vi "Load Signal Bank 1.0.3 keh.vi"(7 "Transpose?":bool, 8 "error in (no error)":errorcluster, 9 "Input array":dbl[][](array[numeric]) format="%.2f", 10 "Active AO Array":u16[](array[numeric]), 11 "timeout (ms)":i32=5000) -> (0 "error out":errorcluster={"status"=FALSE, "code"=0, "source"="."}, 1 "Abort AO":bool, 3 "Time":i32)   [LabVIEW 2020]
uses:
  DAQ Engine VIs/PXI Globals.vi
panel:
  out "Waveform Graph":dbl[][](graph)
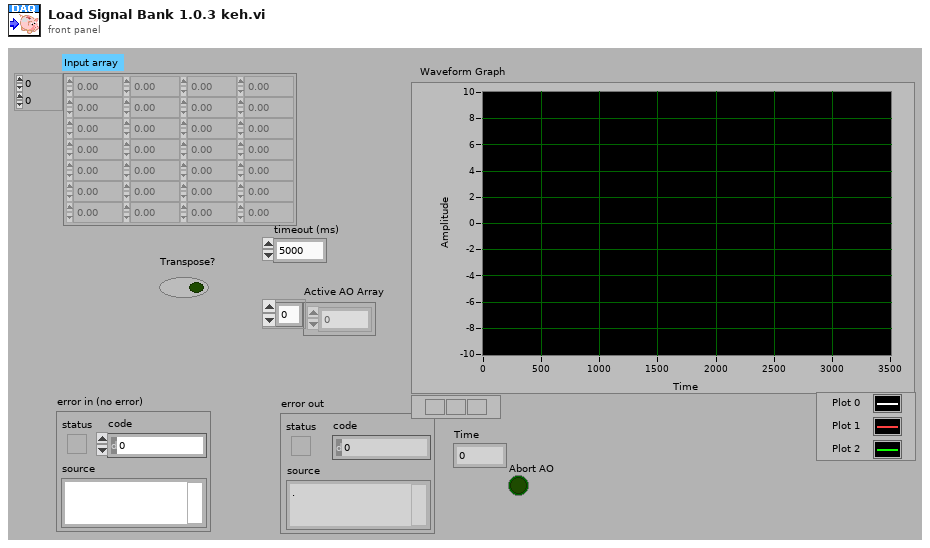
[diagram p1: front panel]
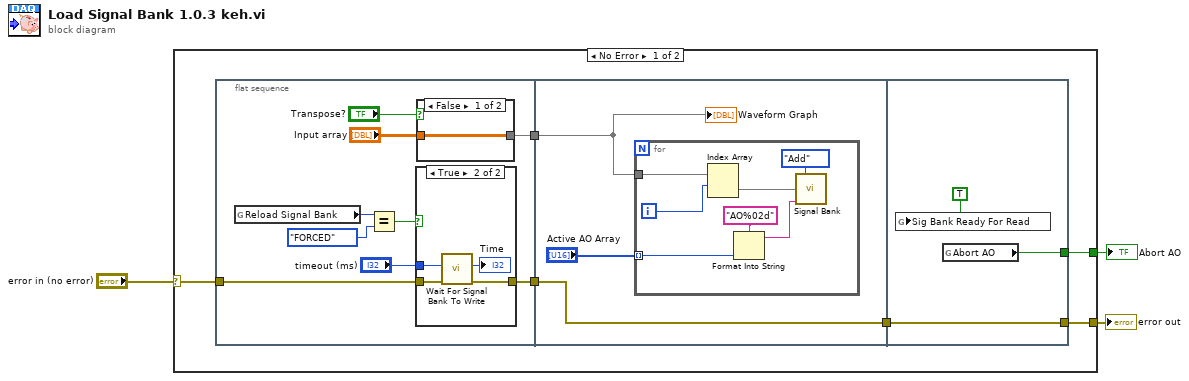
[diagram p0: block diagram]
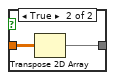
[diagram p2: hidden frame]
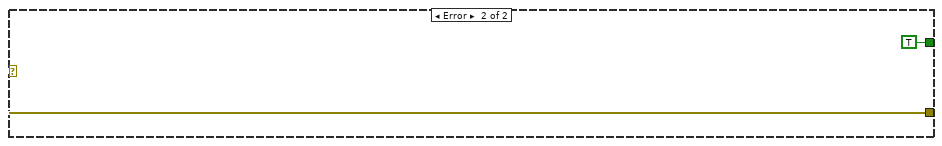
[diagram p4: hidden frame]
diagram:
  n1 = case shown="No Error" "error in (no error)" {
    selector: "error in (no error)" -> [w6 w41]
    tunnel: [w7 w41] -> w3
    tunnel: [w4 TRUE ("Abort AO")] -> w1
    frame No Error {
      n2 = flat-sequence {
        tunnel: w6 -> [w15]
        tunnel: [w18] -> w9
        tunnel: [w10] -> w5
        tunnel: w9 -> [w29]
        tunnel: [w29] -> w8
        tunnel: w5 -> [w27]
        tunnel: [w38] -> w7
        tunnel: w8 -> [w38]
        tunnel: [w37] -> w4
        frame #0 {
          n3 = global read "PXI Globals.vi" "Reload Signal Bank"() -> (w16:enum32{"OFF", "ENABLED", "FORCED"})
          n4 = Equal?(x=w16, y=enum16{"OFF", "ENABLED", "FORCED"}."FORCED") -> (x = y?=w13:bool)
          n5 = case shown="True" w13 {
            tunnel: w15 -> [w22 w26]
            tunnel: [w22 w25] -> w18
            tunnel: "timeout (ms)" -> [_ w24]
            frame False {
            }
            frame True {
              n6 = call "Wait For Signal Bank To Write.vi"("error in (no error)"=w26, "timeout (ms)"=w24) -> ("error out"=w25:errorcluster, "Time"=→"Time":i32)  [unwired: 8 in]
            }
          }
          n7 = case shown="False" "Transpose?" {
            tunnel: "Input array" -> [w19 w21]
            tunnel: [w19 w20] -> w10
            frame False {
            }
            frame True {
              n8 = Transpose 2D Array(2D array=w21) -> (transposed array=w20:dbl[][])
            }
          }
        }
        frame #1 {
          n9 = for {
            tunnel: "Active AO Array" -> [w35] mode=indexing
            tunnel: w27 -> [w30]
            i -> [w33]
            n10 = Index Array(array=w30, index (row)=w33) -> (element=w32:dbl[])  [unwired: 1 in]
            n11 = Format Into String(format string="AO%02d", w35) -> (resulting string=w34:string)  [unwired: 2 in, 1 out]
            n12 = call "Signal Bank.vi"("Action"=enum16{"Add", "Replace ID", "Read ID", "Clear"}."Add", "1D Data In"=w32, "ID"=w34) -> ()  [unwired: 11 in, 2 out]
          }
          "Waveform Graph" <- w27
        }
        frame #2 {
          n13 = global write "PXI Globals.vi" "Sig Bank Ready For Read"(TRUE) -> ()
          n14 = global read "PXI Globals.vi" "Abort AO"() -> (w37:bool)
        }
      }
    }
    frame Error {
    }
  }
  "error out" <- w3
  "Abort AO" <- w1
